vi "power spectrum.vi"() -> ()   [LabVIEW 2017]
uses:
  <instrlib>/niUSRP/niUSRP Fetch Rx Data (CDB WDT).vi
  <vilib>/measure/maspectr.llb/FFT Power Spectrum and PSD for 1 Chan (CDB).vi
  <vilib>/measure/NI_MAPro.lvlib
panel:
  out "coerced IQ rate":dbl=100000.0 format="%#_6p"
  in  "Configuration:Bandwidth":dbl=500000.0 format="%#_13p"
  in  "averaging parameters":T1={"averaging mode"=enum."RMS averaging", "weighting mode"=enum."Exponential", "number of averages"=50} {"number of averages" min=1}
  out "Waveform Graph":cluster{"f0":dbl, "df":dbl, "magnitude":dbl[]}(graph)
  in  "IQ rate":dbl=2500000.0 format="%#_13g"
  in  "gain":dbl=60.0 format="%#_6f"
  in  "device name":refnum<k15>="MyB210"
  in  "freq.":dbl=103900000.0 format="%#_6p"
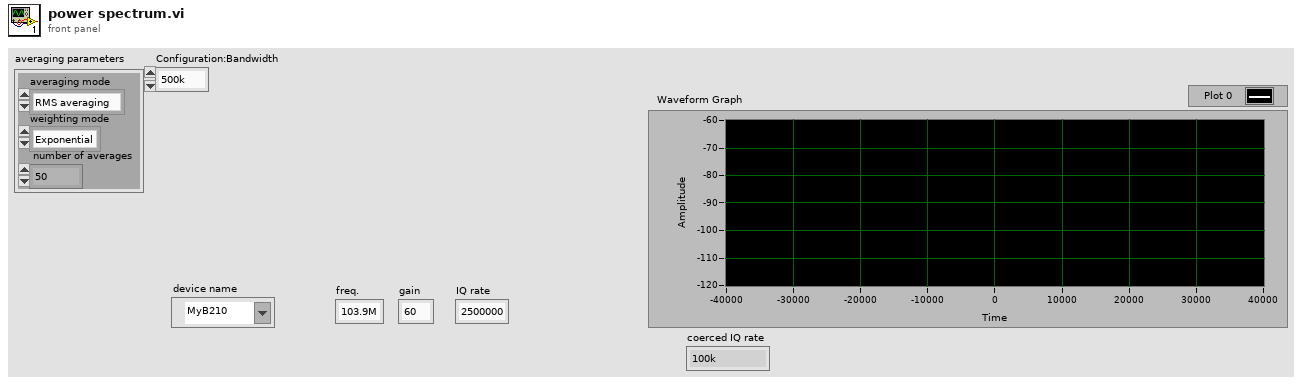
[diagram p1: front panel]
types:
  T1 = cluster{"averaging mode":enum16{"No averaging", "Vector averaging", "RMS averaging", "Peak hold"}, "weighting mode":enum16{"Linear", "Exponential"}, "number of averages":u32}
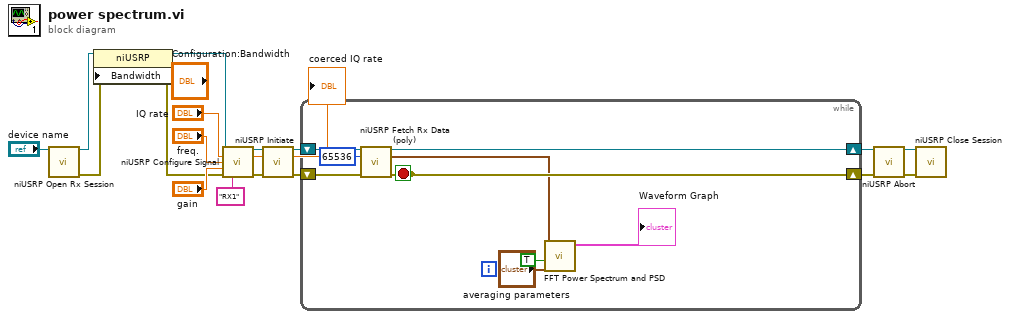
[diagram p0: block diagram]
diagram:
  n1 = call <instrlib>:"niUSRP Open Rx Session.vi"("device names"="device name") -> ("session handle out"=w4:refnum<k15>, "error out"=w5:errorcluster)  [unwired: 13 in]
  n2 = property class="niUSRP"(reference=w4, error in=w5, "Bandwidth"="Configuration:Bandwidth") -> (reference out=w3:refnum<k15>, error out=w2:errorcluster)
  n3 = call <instrlib>:"niUSRP Configure Signal.vi"("session handle"=w3, "IQ rate"="IQ rate", "carrier frequency"="freq.", "gain"="gain", "error in (no error)"=w2, "active antenna"="RX1") -> ("session handle out"=w14:refnum<k15>, "coerced IQ rate"=→"coerced IQ rate":dbl, "error out"=w13:errorcluster)  [unwired: 5 in, 2 out]
  n4 = call <instrlib>:"niUSRP Initiate.vi"("session handle"=w14, "error in (no error)"=w13) -> ("session handle out"=w12:refnum<k15>, "error out"=w11:errorcluster)  [unwired: 12 in]
  n5 = while {
    shift-right: [w27] -> w9
    shift-left: w11 -> [w28]
    shift-right: [w25] -> w7
    shift-left: w12 -> [w26]
    stop <- w27 stop-if-true
    n6 = call-poly <instrlib>:"niUSRP Fetch Rx Data (poly).vi"("session handle"=w26, "number of samples"=65536 ("channel 2"), "error in (no error)"=w28) -> ("session handle out"=w25:refnum<k15>, "data"=w22:waveform(cdb), "error out"=w27:errorcluster)  [unwired: 9 in, 1 out]
    n7 = call-poly <vilib>:"FFT Power Spectrum and PSD.vi"("averaging parameters"="averaging parameters", "dB On (F)"=TRUE, "time signal"=w22) -> ("Power Spectrum / PSD"=→"Waveform Graph":cluster{"f0":dbl, "df":dbl, "magnitude":dbl[]})  [unwired: 5 in, 3 out]
  }
  n8 = call <instrlib>:"niUSRP Abort.vi"("session handle"=w7, "error in (no error)"=w9) -> ("session handle out"=w10:refnum<k15>, "error out"=w8:errorcluster)  [unwired: 12 in]
  n9 = call <instrlib>:"niUSRP Close Session.vi"("session handle"=w10, "error in (no error)"=w8) -> ()  [unwired: 13 in, 1 out]
